vi "TestExec.Control, Select Sequence.vi"(7 "Module Q Name":string, 8 "error in":errorcluster, 10 "Seq":string, 11 "Q In":refnum<queue>) -> (0 "error out":errorcluster, 3 "Q Out":refnum<queue>)   [LabVIEW 2018]
uses:
  <vilib>/KATE/Queues/Q.Element.ctl
  <vilib>/KATE/Queues/Queue Utils.lvlib
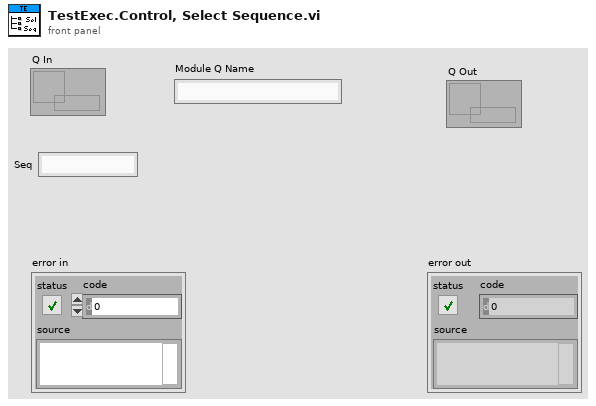
[diagram p1: front panel]
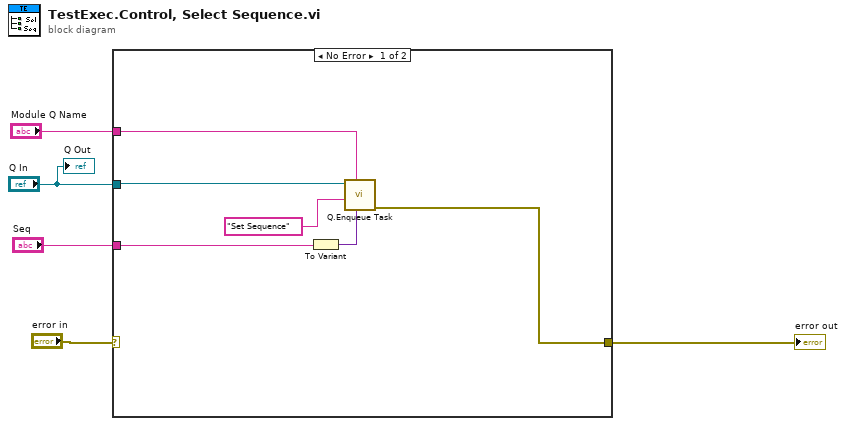
[diagram p0: block diagram]
diagram:
  n1 = case shown="No Error" "error in" {
    selector: "error in" -> [_ w12]
    tunnel: [w7 w12] -> w4
    tunnel: "Q In" -> [w6 _]
    tunnel: "Module Q Name" -> [w9 _]
    tunnel: "Seq" -> [w8 _]
    frame No Error {
      n2 = To Variant(anything=w8) -> (Variant=w11:variant)
      n3 = call <vilib>:"Q.Enqueue Task.vi"("Data1"=w11, "Q Name"=w9, "Task Name"="Set Sequence", "Q In"=w6) -> ("error out"=w7:errorcluster)  [unwired: 6 in, 1 out]
    }
    frame Error {
    }
  }
  "error out" <- w4
  "Q Out" <- "Q In"
